vi "RX Message Queue Ref.vi"(8 "Error In":errorcluster) -> (0 "error out":errorcluster, 3 "rx queue ref":refnum<queue>)   [LabVIEW 2014]
uses:
  Controls/Websocket Data.ctl
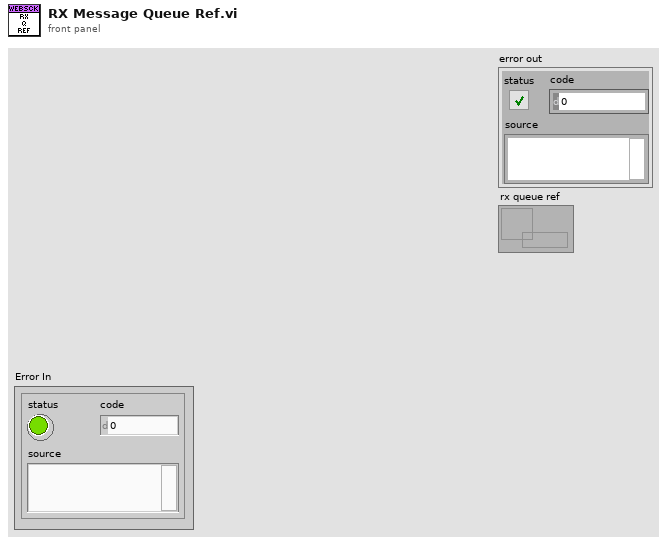
[diagram p1: front panel]
types:
  T1 = typedef "Websocket Data.ctl" = cluster{"Command":string, "Data":string}
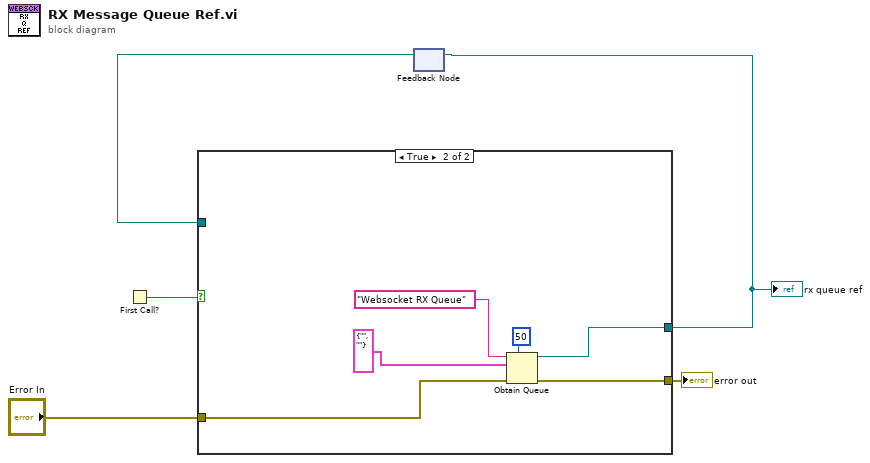
[diagram p0: block diagram]
diagram:
  n1 = First Call?() -> (First Call?: T/F=w5:bool)
  n2 = feedback #1() -> (w2:refnum<queue>)  [unwired: 1 in]
  n3 = case shown="True" w5 {
    tunnel: "Error In" -> [w6 w13]
    tunnel: [w6 w9] -> w1
    tunnel: [w7 w8] -> w3
    tunnel: w2 -> [w7 _]
    frame False {
    }
    frame True {
      n4 = Obtain Queue(max queue size (-1, unlimited)=50, name (unnamed)="Websocket RX Queue", element data type=T1 {"Command"="", "Data"=""} ("Websocket Data"), error in (no error)=w13) -> (queue out=w8:refnum<queue>, error out=w9:errorcluster)  [unwired: 1 in, 1 out]
    }
  }
  "error out" <- w1
  "rx queue ref" <- w3
  n5 = feedback-in #1(w3) -> ()
